vi "Scanned Read - UDV.vi"(5 "FXP VI Ref":refnum<vi>, 7 "UDV Data Type":T2, 8 "error in (no error)":errorcluster, 10 "FXP Config":T1, 11 "IOV ref in":refnum<k21>) -> (0 "error out":errorcluster, 1 "data out":dbl, 3 "IOV ref out":refnum<k21>)   [LabVIEW 2020, in "SEECD Engine.lvlib"]
uses:
  SEECD Engine.lvlib
  Shared/Type Defs/UDV Data Type.ctl
  Shared/Type Defs/FXP Config.ctl
  Shared/SEECD Shared.lvlib
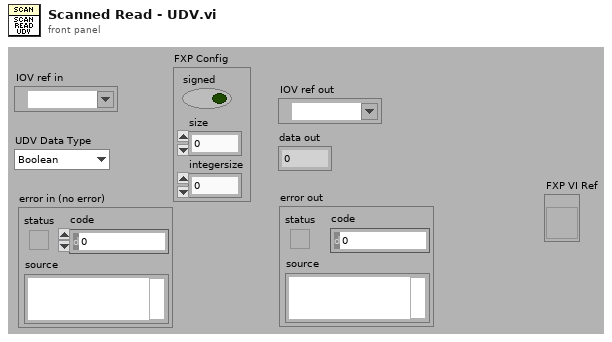
[diagram p1: front panel]
types:
  T1 = typedef "SEECD Shared.lvlib/FXP Config.ctl" = cluster{"signed":bool, "size":u32, "integersize":i32}
  T2 = typedef "SEECD Shared.lvlib/UDV Data Type.ctl" = enum16{"Boolean", "Fixed Point", "Int8", "Int16", "Int32", "Int64", "U32 Bit Field", "UInt8", "UInt16", "UInt32", "UInt64", "Other", "DBL", "SGL"}
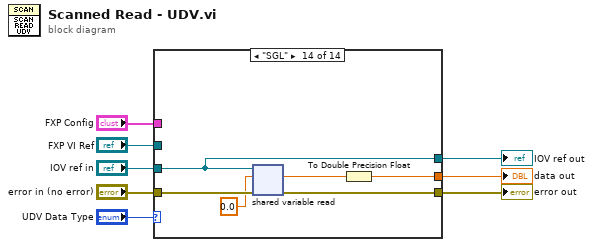
[diagram p0: block diagram]
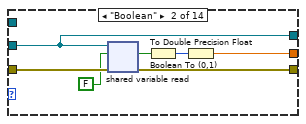
[diagram p3: hidden frame]
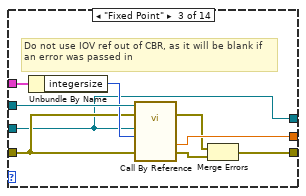
[diagram p4: hidden frame]
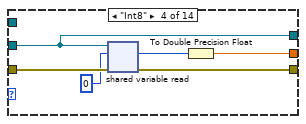
[diagram p5: hidden frame]
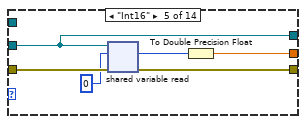
[diagram p6: hidden frame]
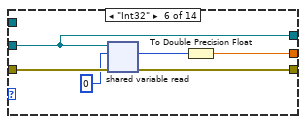
[diagram p7: hidden frame]
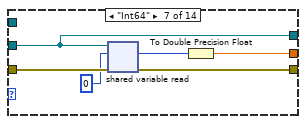
[diagram p8: hidden frame]
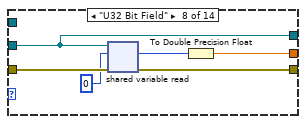
[diagram p9: hidden frame]
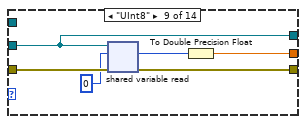
[diagram p10: hidden frame]
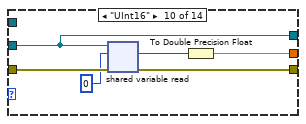
[diagram p11: hidden frame]
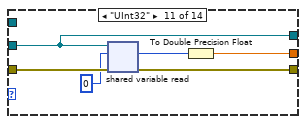
[diagram p12: hidden frame]
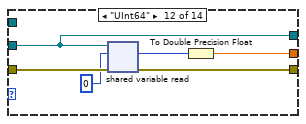
[diagram p13: hidden frame]
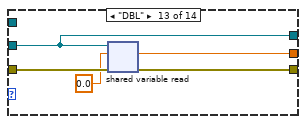
[diagram p14: hidden frame]
diagram:
  n1 = case shown="\"SGL\"" "UDV Data Type" {
    tunnel: "IOV ref in" -> [w10 w14 w18 w30 w36 w42 w48 w54 w60 w66 w72 w78 w83 w89]
    tunnel: [w10 w14 w18 w30 w36 w42 w48 w54 w60 w66 w72 w78 w83 w89] -> w6
    tunnel: "error in (no error)" -> [w9 w17 w23 w32 w38 w44 w50 w56 w62 w68 w74 w80 w85 w91]
    tunnel: [w9 w15 w21 w31 w37 w43 w49 w55 w61 w67 w73 w79 w84 w90] -> w4
    tunnel: "FXP Config" -> [_ _ w25 _ _ _ _ _ _ _ _ _ _ _]
    tunnel: "FXP VI Ref" -> [_ _ w26 _ _ _ _ _ _ _ _ _ _ _]
    tunnel: [_ w11 w22 w29 w35 w41 w47 w53 w59 w65 w71 w77 w81 w86] -> w2
    frame Default {
    }
    frame "Boolean" {
      n2 = shared-variable-read(w14, w17, FALSE) -> (w15:errorcluster, w12:bool)  [unwired: 2 out]
      n3 = Boolean To (0,1)(Boolean=w12) -> (0, 1=w13:i16)
      n4 = To Double Precision Float(number=w13) -> (double precision float=w11:dbl)
    }
    frame "Fixed Point" {
      # "Do not use IOV ref out of CBR, as it will be blank if an error was passed in"
      n5 = Unbundle By Name(w25) -> ("integersize"=w24:i32)
      n6 = call-by-ref "?"(reference=w26, error in=w23, 8:"error in (no error)"=w23, "integersize"=w24, "shared variable refnum in"=w18) -> (error out=w19:errorcluster, 0:"error out"=w20:errorcluster, "data out"=w22:dbl)  [unwired: 6 in, 2 out]
      n7 = Merge Errors(w19, w20) -> (w21:errorcluster)
    }
    frame "Int8" {
      n8 = shared-variable-read(w30, w32, i8 0) -> (w31:errorcluster, w27:i8)  [unwired: 2 out]
      n9 = To Double Precision Float(number=w27) -> (double precision float=w29:dbl)
    }
    frame "Int16" {
      n10 = shared-variable-read(w36, w38, i16 0) -> (w37:errorcluster, w33:i16)  [unwired: 2 out]
      n11 = To Double Precision Float(number=w33) -> (double precision float=w35:dbl)
    }
    frame "Int32" {
      n12 = shared-variable-read(w42, w44, 0) -> (w43:errorcluster, w39:i32)  [unwired: 2 out]
      n13 = To Double Precision Float(number=w39) -> (double precision float=w41:dbl)
    }
    frame "Int64" {
      n14 = shared-variable-read(w48, w50, i64 0) -> (w49:errorcluster, w45:i64)  [unwired: 2 out]
      n15 = To Double Precision Float(number=w45) -> (double precision float=w47:dbl)
    }
    frame "U32 Bit Field" {
      n16 = shared-variable-read(w54, w56, u32 0) -> (w55:errorcluster, w51:u32)  [unwired: 2 out]
      n17 = To Double Precision Float(number=w51) -> (double precision float=w53:dbl)
    }
    frame "UInt8" {
      n18 = shared-variable-read(w60, w62, u8 0) -> (w61:errorcluster, w57:u8)  [unwired: 2 out]
      n19 = To Double Precision Float(number=w57) -> (double precision float=w59:dbl)
    }
    frame "UInt16" {
      n20 = shared-variable-read(w66, w68, u16 0) -> (w67:errorcluster, w63:u16)  [unwired: 2 out]
      n21 = To Double Precision Float(number=w63) -> (double precision float=w65:dbl)
    }
    frame "UInt32" {
      n22 = shared-variable-read(w72, w74, u32 0) -> (w73:errorcluster, w69:u32)  [unwired: 2 out]
      n23 = To Double Precision Float(number=w69) -> (double precision float=w71:dbl)
    }
    frame "UInt64" {
      n24 = shared-variable-read(w78, w80, u64 0) -> (w79:errorcluster, w75:u64)  [unwired: 2 out]
      n25 = To Double Precision Float(number=w75) -> (double precision float=w77:dbl)
    }
    frame "DBL" {
      n26 = shared-variable-read(w83, w85, 0.0) -> (w84:errorcluster, w81:dbl)  [unwired: 2 out]
    }
    frame "SGL" {
      n27 = shared-variable-read(w89, w91, sgl 0.0) -> (w90:errorcluster, w87:sgl)  [unwired: 2 out]
      n28 = To Double Precision Float(number=w87) -> (double precision float=w86:dbl)
    }
  }
  "error out" <- w4
  "IOV ref out" <- w6
  "data out" <- w2
